vi "REFPROP2dll.vi"(8 "error in (no error)":errorcluster, 11 "Inputs":T1) -> (0 "error out":errorcluster, 3 "Outputs":T2)   [LabVIEW 2015]
doc: "subroutine REFPROP2dll(hFld, hIn, hOut, iUnits, iFlag, a, b, z, Output, q, ierr, herr, hFld_length, hIn_length, hOut_length, herr_length)\nShort version of subroutine REFPROP that eliminates the less used variables such as the x and y composition arrays. If the error number (ierr) is zero, the string contained in hUnits will be sent back in herr.\n\nIf q (quality) returns a value between zero and one (and thus the state is two-phase), the REFPROP routine will be needed to obtain the equilibrium compositions.\n\nSee subroutine REFPROP for further information on the input and output variables below.\n\nINPUTS: \nhFld -- Fluid string.\nhIn -- Input string of properties being sent to the routine.\nhOut -- Output string of properties to be calculated.\niUnits -- The unit system to be used for the input and output properties (such as SI, English, etc.)\niFlag -- Flag to specify if the routine SATSPLN should be called (where a value of 1 activates the call).\na -- First input property as specified in the hIn variable.\nb -- Second input property as specified in the hIn variable.\nz -- Molar composition (array of size ncmax=20).\n\nOUTPUTS:\nOutput -- Array of properties specified by the hOut string (array of size 200 dimensioned as double precision). The number -9999970 will be returned when errors occur, and the number -9999990 will be returned when nothing was calculated. Read the comments in the ALLPROPS routine to fully understand the contents of this array.\nq -- Vapor quality on a mole basis.\nierr -- Error flag\nherr -- Error string (character*255)\nhFld_length -- length of variable hFld (default: 10000)\nhIn_length -- length of variable hIn (default: 255)\nhOut_length -- length of variable hOut (default: 255)\nherr_length -- length of variable herr (default: 255)"
uses:
  REFPROP.dll
panel:
  # "REFPROP-REFPROP2dll.vi"
  # "void REFPROP2dll(char *hFld, char *hIn, char *hOut, int *iUnits, int *iFlag, double *a, double *b, double *z/* 20 */, double *Output/* 200 */, double *q, int *ierr, char *herr, int hFld_length/* 10000 */, int hIn_length/* 255 */, int hOut_length/* 255 */, int herr_length/* 255 */);"
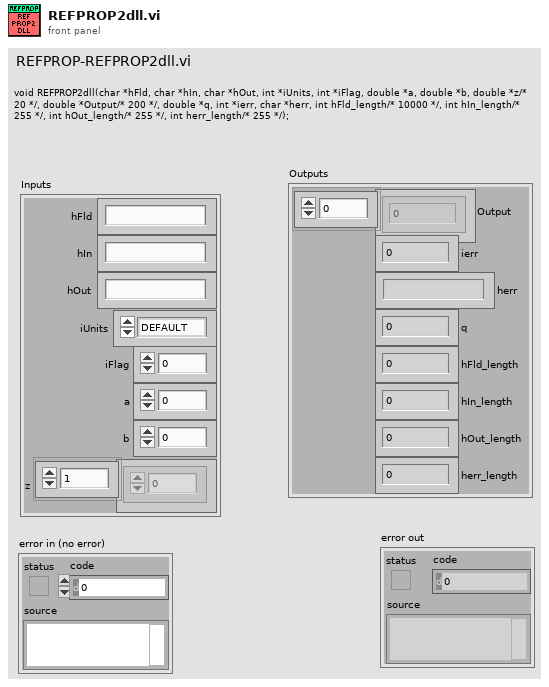
[diagram p1: front panel]
types:
  T1 = cluster{"hFld":string, "hIn":string, "hOut":string, "iUnits":enum32{"DEFAULT", "MOLE SI", "MASS SI", "SI WITH C"}, "iFlag":i32, "a":dbl, "b":dbl, "z":dbl[]}
  T2 = cluster{"Output":dbl[], "ierr":i32, "herr":string, "q":dbl, "hFld_length":i32, "hIn_length":i32, "hOut_length":i32, "herr_length":i32}
  T3 = enum32{"DEFAULT", "MOLE SI", "MASS SI", "SI WITH C"}
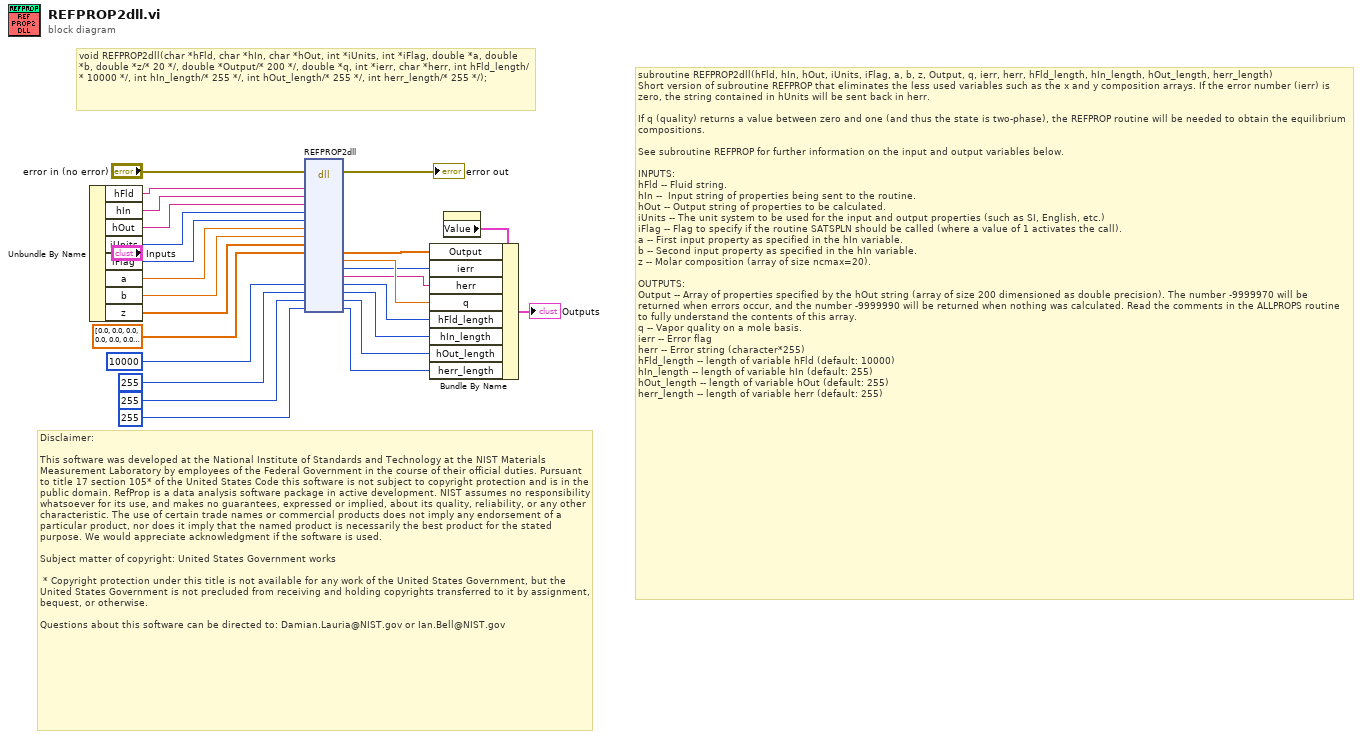
[diagram p0: block diagram]
diagram:
  # "Disclaimer:\n\nThis software was developed at the National Institute of Standards and Technology at the NIST Materials Measurement Laboratory by employees of the Federal Government in the course of their official duties. Pursuant to title 17 section 105* of the United States Code this software is not subject to copyright protection and is in the public domain. RefProp is a data analysis software package in active development. NIST assumes no responsibility whatsoever for its use, and makes no guarantees, expressed or implied, about its quality, reliability, or any other characteristic. The use of certain trade names or commercial products does not imply any endorsement of a particular product, nor does it imply that the named product is necessarily the best product for the stated purpose. We would appreciate acknowledgment if the software is used.\n \nSubject matter of copyright: United States Government works\n  \n * Copyright protection under this title is not available for any work of the United States Government, but the United States Government is not precluded from receiving and holding copyrights transferred to it by assignment, bequest, or otherwise.\n\nQuestions about this software can be directed to: Damian.Lauria@NIST.gov or Ian.Bell@NIST.gov"
  # "subroutine REFPROP2dll(hFld, hIn, hOut, iUnits, iFlag, a, b, z, Output, q, ierr, herr, hFld_length, hIn_length, hOut_length, herr_length)\nShort version of subroutine REFPROP that eliminates the less used variables such as the x and y composition arrays. If the error number (ierr) is zero, the string contained in hUnits will be sent back in herr.\n\nIf q (quality) returns a value between zero and one (and thus the state is two-phase), the REFPROP routine will be needed to obtain the equilibrium compositions.\n\nSee subroutine REFPROP for further information on the input and output variables below.\n\nINPUTS:\t\nhFld -- Fluid string.\nhIn --  Input string of properties being sent to the routine.\nhOut -- Output string of properties to be calculated.\niUnits -- The unit system to be used for the input and output properties (such as SI, English, etc.)\niFlag -- Flag to specify if the routine SATSPLN should be called (where a value of 1 activates the call).\na -- First input property as specified in the hIn variable.\nb -- Second input property as specified in the hIn variable.\nz -- Molar composition (array of size ncmax=20).\n\nOUTPUTS:\nOutput -- Array of properties specified by the hOut string (array of size 200 dimensioned as double precision). The number -9999970 will be returned when errors occur, and the number -9999990 will be returned when nothing was calculated. Read the comments in the ALLPROPS routine to fully understand the contents of this array.\nq -- Vapor quality on a mole basis.\nierr -- Error flag\nherr -- Error string (character*255)\nhFld_length -- length of variable hFld (default: 10000)\nhIn_length -- length of variable hIn (default: 255)\nhOut_length -- length of variable hOut (default: 255)\nherr_length -- length of variable herr (default: 255)"
  # "void REFPROP2dll(char *hFld, char *hIn, char *hOut, int *iUnits, int *iFlag, double *a, double *b, double *z/* 20 */, double *Output/* 200 */, double *q, int *ierr, char *herr, int hFld_length/* 10000 */, int hIn_length/* 255 */, int hOut_length/* 255 */, int herr_length/* 255 */);"
  n1 = Unbundle By Name("Inputs") -> ("hFld"=w24:string, "hIn"=w23:string, "hOut"=w22:string, "iUnits"=w21:T3, "iFlag"=w20:i32, "a"=w19:dbl, "b"=w18:dbl, "z"=w17:dbl[])
  n2 = dll-call lib="C:/Users/lauria/Desktop/REFPROP 10 LabVIEW Wrapper BETA/REFPROP/REFPROP.*" fn="REFPROP2dll"(error in="error in (no error)", "hFld"=w24, "hIn"=w23, "hOut"=w22, "iUnits"=w21, "iFlag"=w20, "a"=w19, "b"=w18, "z"=w17, "Output"=dbl[] [0.0, 0.0, 0.0, 0.0, 0.0, 0.0, 0.0, 0.0, 0.0, 0.0, 0.0, 0.0, 0.0, 0.0, 0.0, 0.0, 0.0, 0.0, 0.0, 0.0, 0.0, 0.0, 0.0, 0.0, 0.0, 0.0, 0.0, 0.0, 0.0, 0.0, 0.0, 0.0, 0.0, 0.0, 0.0, 0.0, 0.0, 0.0, 0.0, 0.0, 0.0, 0.0, 0.0, 0.0, 0.0, 0.0, 0.0, 0.0, 0.0, 0.0, 0.0, 0.0, 0.0, 0.0, 0.0, 0.0, 0.0, 0.0, 0.0, 0.0, 0.0, 0.0, 0.0, 0.0, 0.0, 0.0, 0.0, 0.0, 0.0, 0.0, 0.0, 0.0, 0.0, 0.0, 0.0, 0.0, 0.0, 0.0, 0.0, 0.0, 0.0, 0.0, 0.0, 0.0, 0.0, 0.0, 0.0, 0.0, 0.0, 0.0, 0.0, 0.0, 0.0, 0.0, 0.0, 0.0, 0.0, 0.0, 0.0, 0.0, 0.0, 0.0, 0.0, 0.0, 0.0, 0.0, 0.0, 0.0, 0.0, 0.0, 0.0, 0.0, 0.0, 0.0, 0.0, 0.0, 0.0, 0.0, 0.0, 0.0, 0.0, 0.0, 0.0, 0.0, 0.0, 0.0, 0.0, 0.0, 0.0, 0.0, 0.0, 0.0, 0.0, 0.0, 0.0, 0.0, 0.0, 0.0, 0.0, 0.0, 0.0, 0.0, 0.0, 0.0, 0.0, 0.0, 0.0, 0.0, 0.0, 0.0, 0.0, 0.0, 0.0, 0.0, 0.0, 0.0, 0.0, 0.0, 0.0, 0.0, 0.0, 0.0, 0.0, 0.0, 0.0, 0.0, 0.0, 0.0, 0.0, 0.0, 0.0, 0.0, 0.0, 0.0, 0.0, 0.0, 0.0, 0.0, 0.0, 0.0, 0.0, 0.0, 0.0, 0.0, 0.0, 0.0, 0.0, 0.0, 0.0, 0.0, 0.0, 0.0, 0.0, 0.0, 0.0, 0.0, 0.0, 0.0, 0.0, 0.0], "hFld_length"=10000, "hIn_length"=255, "hOut_length"=255, "herr_length"=255) -> (error out=→"error out":errorcluster, "Output"=w8:dbl[], "q"=w10:dbl, "ierr"=w9:i32, "herr"=w7:string, "hFld_length"=w11:i32, "hIn_length"=w12:i32, "hOut_length"=w13:i32, "herr_length"=w14:i32)  [unwired: 14 in, 1 out]
  n3 = property on="Outputs" class="Clust (strict)"() -> ("Value"=w16:T2)  [unwired: 2 in, 2 out]
  n4 = Bundle By Name(cluster=w16, "Output"=w8, "ierr"=w9, "herr"=w7, "q"=w10, "hFld_length"=w11, "hIn_length"=w12, "hOut_length"=w13, "herr_length"=w14) -> (→"Outputs":T2)
